vi "Execution Profiler View.vi"(8 "error in (no error)":errorcluster, 11 "Execution Profiler Result View":refnum<class "Execution Profiler Result View.lvclass">) -> (0 "error out":errorcluster)   [LabVIEW 2020, in "Execution Profiler Result View.lvclass"]
uses:
  Execution Profiler Result View/Execution Profiler Result View.lvclass
  Execution Profiler Result View/Execution Profiler Result View.lvclass/Execution Profiler Result View.ctl
  Helper Classes/Open Test Case Interface/Open Test Case.lvclass
panel:
  in  "Method Test Times":i32(listbox)
  out "Histogram":cluster{"X":dbl, "Y":dbl}[](graph)
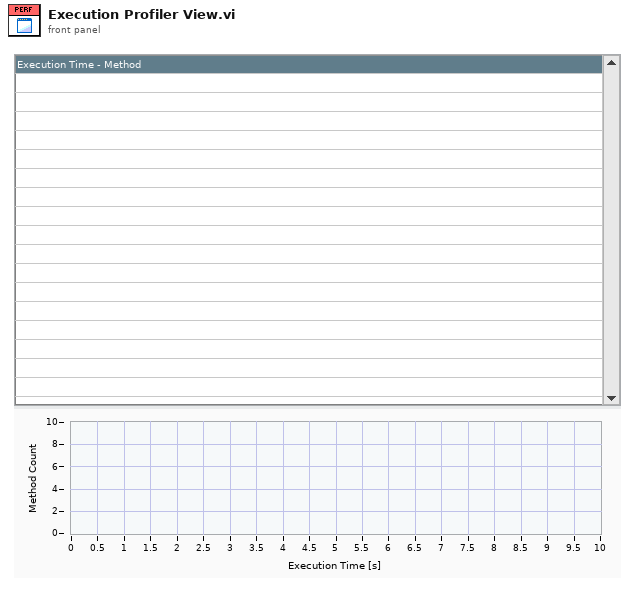
[diagram p1: front panel]
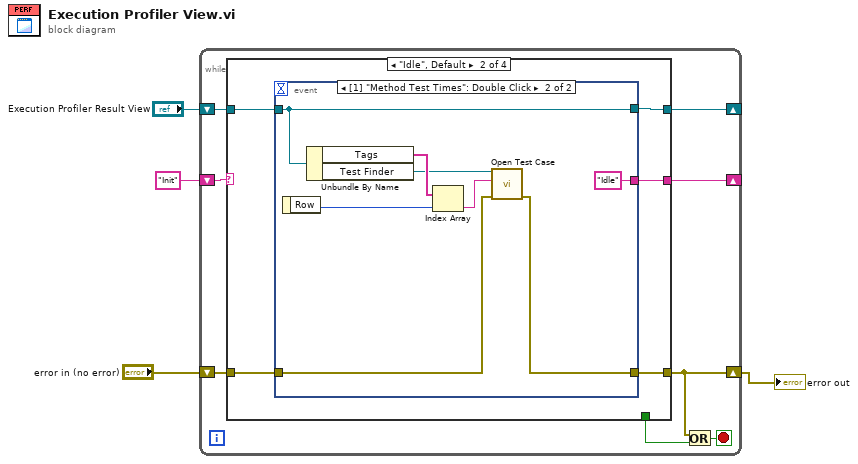
[diagram p0: block diagram]
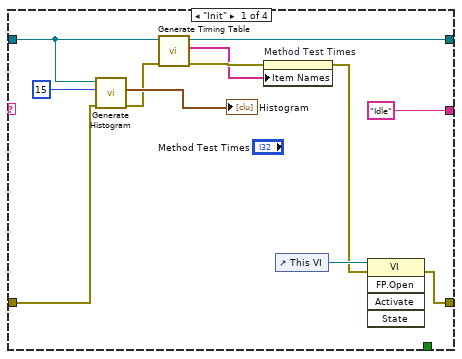
[diagram p2: hidden frame]
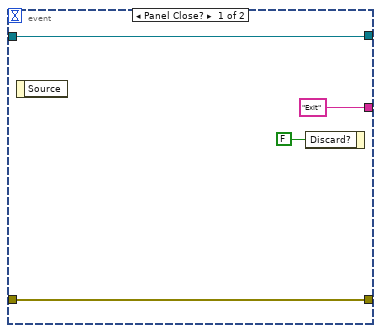
[diagram p3: hidden frame]
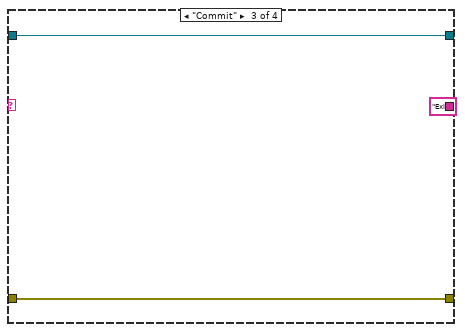
[diagram p4: hidden frame]
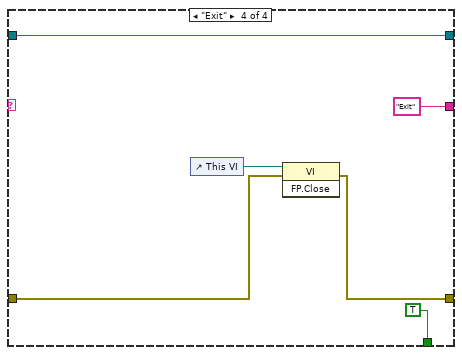
[diagram p5: hidden frame]
diagram:
  n1 = while {
    shift-right: [w9] -> _
    shift-left: "Execution Profiler Result View" -> [w10]
    shift-right: [w5] -> w2
    shift-left: "error in (no error)" -> [w11]
    shift-right: [w8] -> _
    shift-left: "Init" -> [w12]
    stop <- w6 stop-if-true
    n2 = case shown="\"Idle\", Default" w12 {
      tunnel: [w19 w29 w44 w46] -> w5
      tunnel: w11 -> [w22 w28 w44 w45]
      tunnel: w10 -> [w13 w27 w43 w50]
      tunnel: [w18 w26 w43 w50] -> w9
      tunnel: ["Idle" w25 "Exit" "Exit"] -> w8
      tunnel: [_ _ _ TRUE] -> w7
      frame "Init" {
        n3 = call "Generate Histogram.vi"("error in (no error)"=w22, "Interval Scaling"=u8 15 ("Number of intervals"), "View In"=w13) -> ("error out"=w17:errorcluster, "Histogram"=→"Histogram":cluster{dbl, dbl}[])  [unwired: 7 in]
        n4 = call "Generate Timing Table.vi"("error in (no error)"=w17, "Performance Analyzer In"=w13) -> ("error out"=w16:errorcluster, "Timing List"=w14:string[], "Performance Analyzer Out"=w18:refnum<class "Execution Profiler Result View.lvclass">)  [unwired: 7 in]
        n5 = property on="Method Test Times" class="LstBox (strict)"(error in=w16, "Item Names"=w14) -> (error out=w15:errorcluster)  [unwired: 1 in, 1 out]
        n6 = control-ref of="This VI"() -> (w20:refnum<vi>)
        n7 = invoke class="VI" method="FP.Open"(reference=w20, error in=w15) -> (error out=w19:errorcluster)  [unwired: 3 in, 4 out]
      }
      frame "Idle", Default {
        n8 = event shown="[1] \"Method Test Times\": Double Click" {
          selector: _ -> [_ _]
          dyn-events: _ -> [_ _]
          timeout: _ -> [_ _]
          tunnel: [w33 w35] -> w29
          tunnel: w28 -> [w33 w34]
          tunnel: w27 -> [w32 w41]
          tunnel: [w32 w41] -> w26
          tunnel: ["Exit" "Idle"] -> w25
          event Panel Close? {
            n9 = event-data() -> ()  [unwired: 1 in, 1 out]
            n10 = event-data("Discard?"=FALSE) -> ()  [unwired: 1 in, 1 out]
          }
          event "Method Test Times": Double Click {
            n11 = event-data() -> ("Row"=w39:i32)  [unwired: 1 in]
            n12 = Unbundle By Name(w41) -> ("Tags"=w40:string[], "Test Finder"=w37:refnum<class "Open Test Case.lvclass">)
            n13 = Index Array(array=w40, index=w39) -> (element=w36:string)
            n14 = call-dynamic "Open Test Case.vi"("error in (no error)"=w34, "Tag"=w36, "Open Test Case in"=w37) -> ("error out"=w35:errorcluster)  [unwired: 6 in, 2 out]
          }
        }
      }
      frame "Commit" {
      }
      frame "Exit" {
        n15 = control-ref of="This VI"() -> (w47:refnum<vi>)
        n16 = invoke class="VI" method="FP.Close"(reference=w47, error in=w45) -> (error out=w46:errorcluster)  [unwired: 1 in, 2 out]
      }
    }
    n17 = Or(x=w5, y=w7) -> (x .or. y?=w6:bool)
  }
  "error out" <- w2
